vi "checkin.vi"(8 "error in (no error)":errorcluster, 11 "GenericStage in":refnum<class "GenericStage.lvclass">) -> (0 "error out":errorcluster, 3 "GenericStage out":refnum<class "GenericStage.lvclass">)   [LabVIEW 2010, in "GenericStage.lvclass"]
uses:
  GenericStage.lvclass
  common/classes/GenericToplevelComponent/GenericToplevelComponent/GenericToplevelComponent.lvclass
  class_data.vi
  common/classes/ErrorController/ErrorController/class_data.vi
  common/classes/GenericComponent/GenericComponent/GenericComponent.lvclass
  common/classes/ErrorController/ErrorController/ErrorController.lvclass
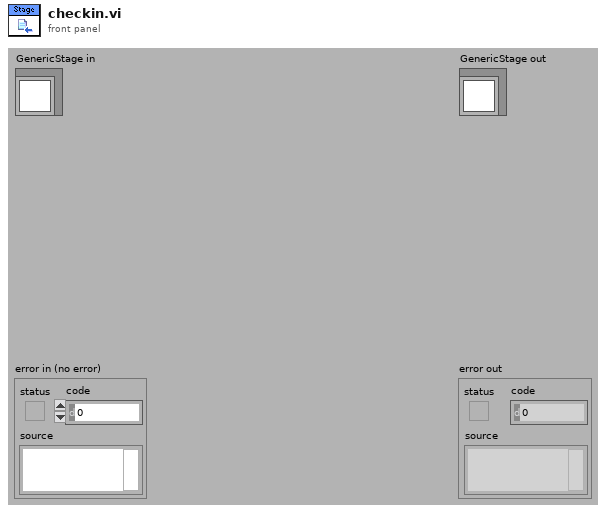
[diagram p1: front panel]
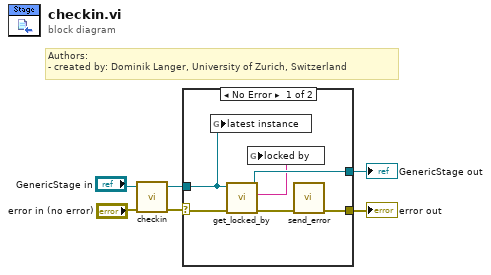
[diagram p0: block diagram]
diagram:
  # "Authors: \n- created by: Dominik Langer, University of Zurich, Switzerland"
  n1 = call-parent "checkin.vi"("error in (no error)"="error in (no error)", "GenericPlugin in"="GenericStage in") -> ("error out"=w1:errorcluster, "GenericPlugin out"=w2:refnum<class "GenericStage.lvclass">)  [unwired: 8 in]
  n2 = case shown="No Error" w1 {
    selector: w1 -> [w8 w14]
    tunnel: [w9 w14] -> w6
    tunnel: [w12 w13] -> w5
    tunnel: w2 -> [w7 w13]
    frame No Error {
      n3 = global write "class_data.vi" "latest instance"(w7) -> ()
      n4 = call "get_locked_by.vi"("error in (no error)"=w8, "GenericPlugin.lvclass in"=w7) -> ("error out"=w10:errorcluster, "locked by"=w11:string, "GenericPlugin.lvclass out"=w12:refnum<class "GenericStage.lvclass">)  [unwired: 7 out]
      n5 = global write "class_data.vi" "locked by"(w11) -> ()
      n6 = call "send_error.vi"("error in (no error)"=w10) -> ("error out"=w9:errorcluster)  [unwired: 10 in]
    }
    frame Error {
    }
  }
  "error out" <- w6
  "GenericStage out" <- w5
